vi "write_fifo_resonance_toggle.vi"(5 "enable fly-back reversion?":bool, 6 "invert channels":bool[](array[boolean])=[FALSE, FALSE], 7 "fly-back?":bool, 8 "pixel finished?":bool, 9 "ch0-ch1?":bool, 10 "maximum bit depth":i8, 11 "integration cluster in":T1) -> (0 "FIFO overflow out":bool, 3 "integration cluster out":T1)   [LabVIEW 2010]
uses:
  integration_cluster.ctl
  <vilib>/rvi/DataTransferAndStorage/Container/XNode/niFpgaContainer.xnode
  <vilib>/rvi/DataTransferAndStorage/Container/Common/niFpgaContainerMethod.ctl
  <vilib>/rvi/DataTransferAndStorage/Container/Common/niFpgaTransferTypeControl.ctl
  <vilib>/rvi/Memory/Memory_Emulation/nirvimemoryEmulationManagerCache_GetValue.vi
  <vilib>/rvi/DataTransferAndStorage/Container/Common/niFpgaContainerGetUniqueNameForEmu.vi
  <vilib>/rvi/Memory/Memory_Emulation/nirvimemoryEmulationManagerCache_InsertValue.vi
  <vilib>/Utility/error.llb/Clear Errors.vi
  <vilib>/rvi/Memory/Memory_Emulation/nirvimemoryEmulationManagerCache_SetValue.vi
  <vilib>/rvi/interface/RandomDataEmulation/nirviRandomDataFPGAFIFO.vi
  <vilib>/rvi/interface/RandomDataEmulation/niFpgaRandomDataHandleErrors.vi
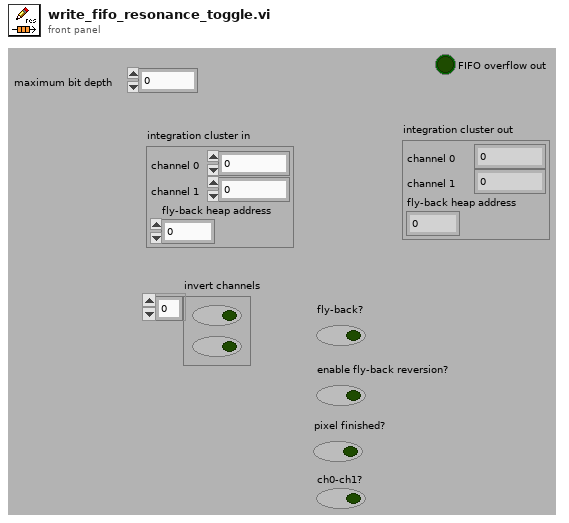
[diagram p1: front panel]
types:
  T1 = typedef "integration_cluster.ctl" = cluster{"channel 0":u32, "channel 1":u32, "fly-back heap address":u32}
  T2 = typedef "niFpgaContainerMethod.ctl" = enum16{"<none>", "write", "read", "clear", "getNumberOfElementsToWrite", "getNumberOfElementsToRead", "enable", "disable", "flushAndDisable", "getStreamState", "readA", "readB", "dramWrite", "dramWriteWithByteEnables", "dramRequestData", "dramRetrieveData"}
  T3 = typedef "niFpgaTransferTypeControl.ctl" = enum16{"Target-Scoped", "Host to Target - DMA", "Target to Host - DMA", "Peer to Peer Reader", "Peer to Peer Writer", "Bidirectional"}
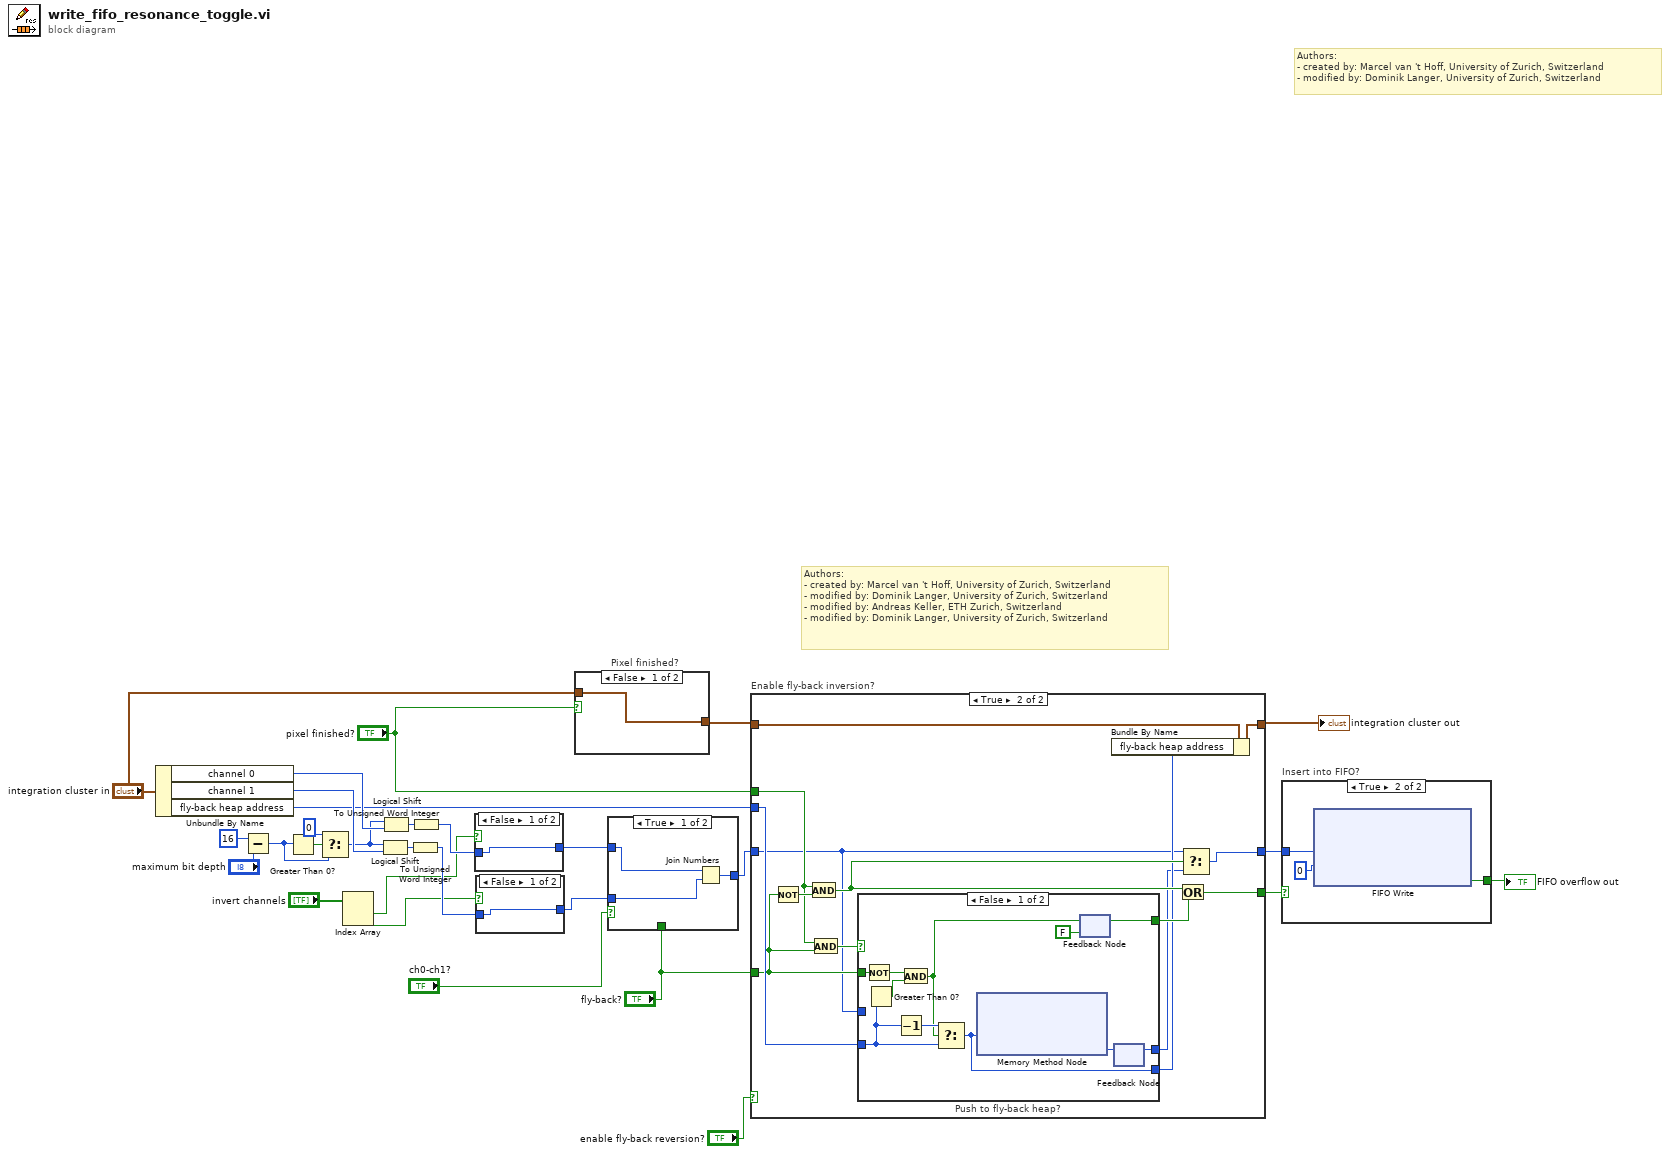
[diagram p0: block diagram]
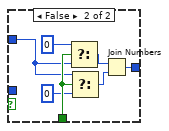
[diagram p2: hidden frame]
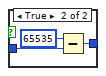
[diagram p3: hidden frame]
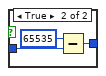
[diagram p4: hidden frame]
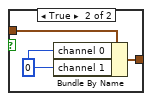
[diagram p5: hidden frame]
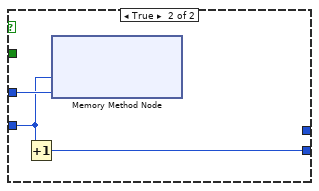
[diagram p7: hidden frame]
diagram:
  # "Authors: \n- created by: Marcel van 't Hoff, University of Zurich, Switzerland\n- modified by: Dominik Langer, University of Zurich, Switzerland\n- modified by: Andreas Keller, ETH Zurich, Switzerland\n- modified by: Dominik Langer, University of Zurich, Switzerland"
  # "Authors: \n- created by: Marcel van 't Hoff, University of Zurich, Switzerland\n- modified by: Dominik Langer, University of Zurich, Switzerland"
  n1 = Unbundle By Name("integration cluster in") -> ("channel 0"=w22:u32, "channel 1"=w23:u32, "fly-back heap address"=w16:u32)
  n2 = Subtract(x=i8 16, y="maximum bit depth") -> (x-y=w25:i8)
  n3 = Greater Than 0?(x=w25) -> (x > 0?=w24:bool)
  n4 = Select(t=i8 0 ("f"), s=w24, f=w25) -> (s? t:f=w21:i8)
  n5 = Index Array(array="invert channels") -> (element #1=w7:bool, element #2=w6:bool)  [unwired: 2 in]
  n6 = Logical Shift(y=w21, x=w23) -> (x << y=w20:u32)
  n7 = Logical Shift(y=w21, x=w22) -> (x << y=w19:u32)
  n8 = To Unsigned Word Integer(number=w20) -> (unsigned 16bit integer=w9:u16)
  n9 = To Unsigned Word Integer(number=w19) -> (unsigned 16bit integer=w10:u16)
  n10 = case shown="False" w7 {
    tunnel: [w30 w32] -> w4
    tunnel: w10 -> [w30 w31]
    frame False {
    }
    frame True {
      n11 = Subtract(x=u16 65535, y=w31) -> (x-y=w32:u16)
    }
  }
  n12 = case shown="False" w6 {
    tunnel: [w34 w36] -> w2
    tunnel: w9 -> [w34 w35]
    frame False {
    }
    frame True {
      n13 = Subtract(x=u16 65535, y=w35) -> (x-y=w36:u16)
    }
  }
  n14 = case "Pixel finished?" shown="False" "pixel finished?" {
    tunnel: "integration cluster in" -> [w38 w40]
    tunnel: [w38 w39] -> w13
    frame False {
    }
    frame True {
      w41 = u32 0 ("channel 1")
      n15 = Bundle By Name(cluster=w40, "channel 0"=w41, "channel 1"=w41) -> (w39:T1)
    }
  }
  n16 = case shown="True" "ch0-ch1?" {
    tunnel: "fly-back?" -> [_ w50]
    tunnel: w4 -> [w43 w48]
    tunnel: [w44 w46] -> w3
    tunnel: w2 -> [w42 _]
    frame True {
      n17 = Join Numbers(hi=w43, lo=w42) -> ((hi.lo)=w44:u32)
    }
    frame False {
      n18 = Select(t=u16 0 ("x"), s=w50, f=w48) -> (s? t:f=w51:u16)
      n19 = Select(t=w48, s=w50, f=u16 0 ("x")) -> (s? t:f=w49:u16)
      n20 = Join Numbers(hi=w51, lo=w49) -> ((hi.lo)=w46:u32)
    }
  }
  n21 = case "Enable fly-back inversion?" shown="True" "enable fly-back reversion?" {
    tunnel: w16 -> [_ w68]
    tunnel: w3 -> [w54 w57]
    tunnel: [w54 w66] -> w18
    tunnel: "pixel finished?" -> [w53 w61]
    tunnel: [w53 w56] -> w15
    tunnel: "fly-back?" -> [_ w63]
    tunnel: w13 -> [w52 w60]
    tunnel: [w52 w58] -> w11
    frame False {
    }
    frame True {
      n22 = Not(x=w63) -> (.not. x?=w67:bool)
      n23 = And(x=w61, y=w67) -> (x .and. y?=w64:bool)
      n24 = And(x=w61, y=w63) -> (x .and. y?=w65:bool)
      n25 = case "Push to fly-back heap?" shown="False" w65 {
        tunnel: w57 -> [_ w208]
        tunnel: [w71 w207] -> w59
        tunnel: w68 -> [w73 w206]
        tunnel: w63 -> [w78 _]
        tunnel: [w75 _] -> w55
        tunnel: [w77 _] -> w62
        frame False {
          n26 = Not(x=w78) -> (.not. x?=w70:bool)
          n27 = Greater Than 0?(x=w73) -> (x > 0?=w79:bool)
          n28 = Decrement(x=w73) -> (x-1=w72:u32)
          n29 = And(x=w70, y=w79) -> (x .and. y?=w69:bool)
          n30 = Select(t=w72, s=w69, f=w73) -> (s? t:f=w71:u32)
          n31 = xnode ("Memory Method Node")("Address"=w71) -> ("Data"=w74:u32)  [unwired: 1 in, 1 out]
          n32 = feedback #1(FALSE) -> (w77:bool)
          n33 = feedback-in #1(w69) -> ()
          n34 = feedback #2() -> (w75:u32)  [unwired: 1 in]
          n35 = feedback-in #2(w74) -> ()
        }
        frame True {
          n36 = Increment(x=w206) -> (x+1=w207:u32)
          n37 = xnode ("Memory Method Node")("Address"=w206, "Data"=w208) -> ()  [unwired: 1 in, 1 out]
        }
      }
      n38 = Bundle By Name(cluster=w60, "fly-back heap address"=w59) -> (w58:T1)
      n39 = Or(x=w64, y=w62) -> (x .or. y?=w56:bool)
      n40 = Select(t=w57, s=w64, f=w55) -> (s? t:f=w66:u32)
    }
  }
  "integration cluster out" <- w11
  n41 = case "Insert into FIFO?" shown="True" w15 {
    tunnel: [_ w336] -> w28
    tunnel: w18 -> [_ w334]
    frame False {
    }
    frame True {
      n42 = xnode ("FIFO Write")("Element"=w334, "Timeout"=0) -> ("Timed Out?"=w336:bool)  [unwired: 1 in, 1 out]
    }
  }
  "FIFO overflow out" <- w28
